vi "LabVIEW_Read_Soil_Moisture.vi"() -> ()   [LabVIEW 2020]
uses:
  <vilib>/Instr/_visa.llb/Select Event Type.ctl
  <vilib>/Instr/_visa.llb/VISA Configure Serial Port (Instr).vi
panel:
  in  "Stop":bool
  in  "Tab Control":T1(tab)
  out "Serial Read Buffer":string
  in  "VISA resource name":refnum<visa-resource-name>="COM17"
  in  "baud rate (9600)":u32=9600
  out "Voltage of Soil Moisture Sensor Chart":dbl(graph)
  out "Reading Rate (ms)":u32
  # "Soil Moisture Read with Arduino and LabVIEW"
  # "Auther: Suparat Yeamkuan\nOverview: Demonstrates the use of Arduino read a voltage from soil moisture sensor to LabVIEW.\nRequirements: Arduino UNO, Soli moisture sensor, and  NI-VISA Driver."
  # "Instructions:\n1. Wiring soil moisture sensor to Arduino board follow below:"
  # "Instructions:\n1. Connect USB cable from Arduino board to computer.\n2. Use Arduino IDE to upload the code to Arduino board."
  # "Instructions:\n1. Select the VISA resource name as a COM port that Arduino connect to computer, this can show the COM port device manager.\n2. Run the VI.\n3. If your Arduino is reading voltage from sensor, it should show a response in the \"Serial Read Buffer\" and Voltage of Soil Moisture Sensor Chart."
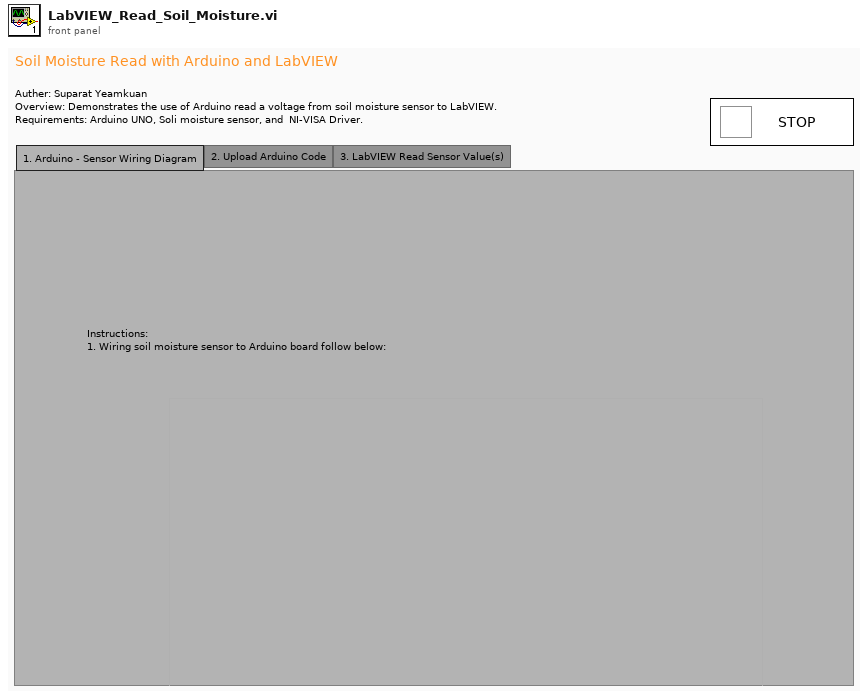
[diagram p1: front panel]
types:
  T1 = enum32{"1. Arduino - Sensor Wiring Diagram", "2. Upload Arduino Code", "3. LabVIEW Read Sensor Value(s)"}
  T2 = typedef "Select Event Type.ctl" = u32
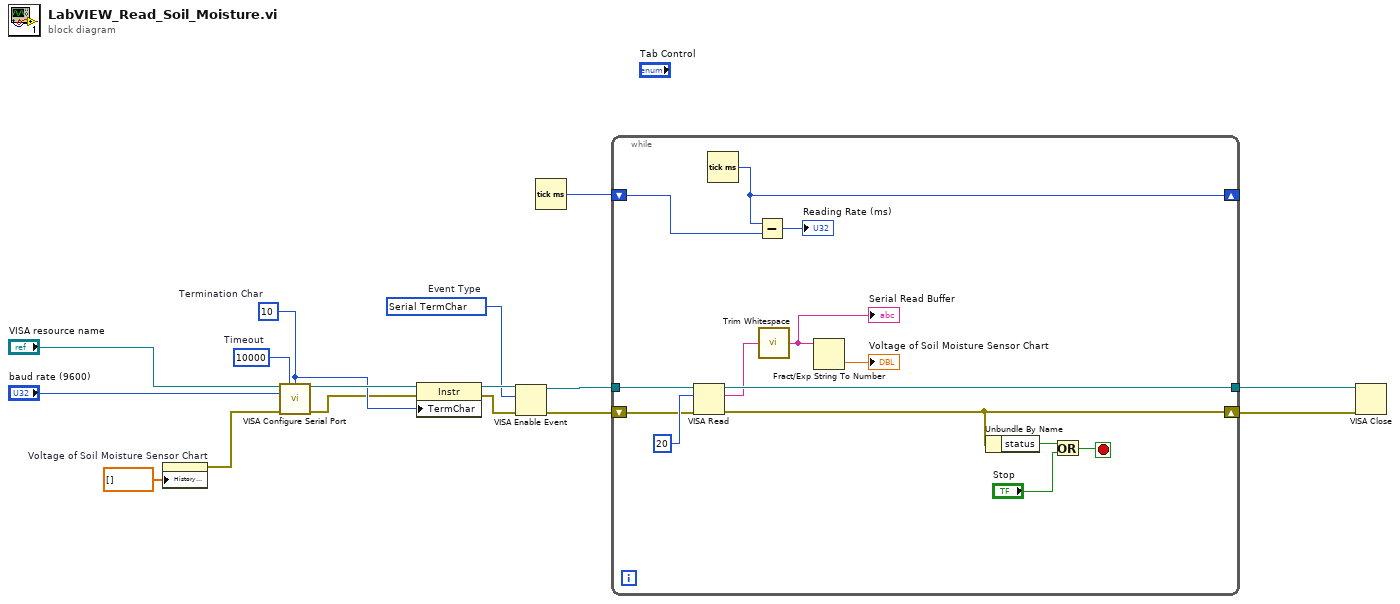
[diagram p0: block diagram]
diagram:
  w8 = T2 1073684516 items=["Service Request"=1073684491, "Trigger"=3221168138, "Clear"=1073684493, "VXI Signal"=1073684512, "VXI/VME Interrupt"=3221168161, "VXI/VME Sysfail"=1073684509, "VXI/VME Sysreset"=1073684510, "GPIB CIC"=1073684498, "GPIB Talk"=1073684499, "GPIB Listen"=1073684500, "PXI Interrupt"=1073684514, "Serial Break"=1073684515, "Serial TermChar"=1073684516, "Serial CTS"=1073684521, "Serial DSR"=1073684522, "Serial DCD"=1073684524, "Serial RI"=1073684526, "Serial Character"=1073684533, "USB Interrupt"=1073684535, "All Enabled"=1073709055]  # Event Type
  w12 = u8 10  # Termination Char
  w14 = u32 10000  # Timeout
  n1 = property on="Voltage of Soil Moisture Sensor Chart" class="WFChart (strict)"("History Data"=dbl[] []) -> (error out=w2:errorcluster)  [unwired: 2 in, 1 out]
  n2 = call-poly "VISA Configure Serial Port"("VISA resource name"="VISA resource name", "timeout (10sec)"=w14, "termination char\n(0xA = '\\n' = LF)"=w12, "baud rate (9600)"="baud rate (9600)", "error in (no error)"=w2) -> ("VISA resource name out"=w13:refnum<visa-resource-name>, "error out"=w11:errorcluster)  [unwired: 9 in]
  n3 = property class="Instr"(reference=w13, error in=w11, "TermChar"=w12) -> (reference out=w10:refnum<visa-resource-name>, error out=w9:errorcluster)
  n4 = VISA Enable Event(8:w9, 10:w8, 11:w10) -> (0:w7:errorcluster, 3:w6:refnum<visa-resource-name>)  [unwired: 1 in]
  n5 = Tick Count (ms)() -> (millisecond timer value=w1:u32)
  n6 = while {
    shift-right: [w29] -> w15
    shift-left: w7 -> [w24]
    tunnel: [w30] -> w16
    tunnel: w6 -> [w23]
    shift-right: [w19] -> _
    shift-left: w1 -> [w18]
    stop <- w27 stop-if-true
    n7 = VISA Read(VISA resource name=w23, byte count=u32 20, error in (no error)=w24) -> (VISA resource name out=w30:refnum<visa-resource-name>, read buffer=w22:string, error out=w29:errorcluster)  [unwired: 1 out]
    n8 = Tick Count (ms)() -> (millisecond timer value=w19:u32)
    n9 = Subtract(x=w19, y=w18) -> (x-y=→"Reading Rate (ms)":u32)
    n10 = call <vilib>:"Trim Whitespace.vi"("string"=w22) -> ("trimmed string"=w21:string)  [unwired: 1 in]
    "Serial Read Buffer" <- w21
    n11 = Fract/Exp String To Number(string=w21) -> (number=→"Voltage of Soil Moisture Sensor Chart":dbl)  [unwired: 3 in, 1 out]
    n12 = Unbundle By Name(w29) -> ("status"=w28:bool)
    n13 = Or(x=w28, y="Stop") -> (x .or. y?=w27:bool)
  }
  n14 = VISA Close(VISA resource name=w16, error in (no error)=w15) -> ()  [unwired: 1 out]
